vi "HFRR ADV v10.vi"() -> ()   [LabVIEW 2025] (continued)
              n2118 = Fract/Exp String To Number(string=w2526) -> (number=w2523:dbl)  [unwired: 3 in, 1 out]
              n2119 = Add(x=w2523, y=0.0) -> (x+y=w2521:dbl)
            }
            n2120 = String To Path(string=w2366) -> (path=w2464:path)
            n2121 = String To Path(string=w2364) -> (path=w2458:path)
            n2122 = local read "Numeric 11"() -> (w2448:i32)
            n2123 = local read "Numeric 13"() -> (w2450:i32)
            n2124 = Open/Create/Replace File "Open File"(file path (use dialog)=w2464) -> (refnum out=w2462:refnum<file>, error out=w2461:errorcluster)  [unwired: 5 in, 1 out]
            n2125 = Open/Create/Replace File "Open File"(file path (use dialog)=w2458) -> (refnum out=w2457:refnum<file>, error out=w2456:errorcluster)  [unwired: 5 in, 1 out]
            n2126 = for {
              N: w2448 -> [_]
              tunnel: w2462 -> [w2577]
              tunnel: w2461 -> [w2576]
              tunnel: [w2566] -> w2428 mode=indexing
              tunnel: [w2564] -> w2426 mode=indexing
              tunnel: [w2565] -> w2421 mode=indexing
              tunnel: w2447 -> [_]
              tunnel: [w2558] -> w2423 mode=indexing
              tunnel: [w2554] -> w2399 mode=indexing
              tunnel: [w2550] -> w2374 mode=indexing
              tunnel: [w2546] -> w2355 mode=indexing
              tunnel: [w2541] -> w2313 mode=indexing
              (unwired) TRUE ("line mode (F)")
              n2127 = Read from Text File "Read File"(file (use dialog)=w2577, error in=w2576) -> (text=w2542:string)  [unwired: 2 in, 3 out]
              n2128 = local write "String 7"(w2542) -> ()
              n2129 = String Subset(string=w2542, offset (0)=85, length (rest)=9 ("length (rest)")) -> (substring=w2545:string)
              n2130 = String Subset(string=w2542, offset (0)=35, length (rest)=9 ("length (rest)")) -> (substring=w2567:string)
              n2131 = String Subset(string=w2542, offset (0)=55, length (rest)=9 ("length (rest)")) -> (substring=w2553:string)
              n2132 = String Subset(string=w2542, offset (0)=25, length (rest)=9 ("length (rest)")) -> (substring=w2547:string)
              n2133 = String Subset(string=w2542, offset (0)=45, length (rest)=9 ("length (rest)")) -> (substring=w2555:string)
              n2134 = String Subset(string=w2542, offset (0)=0, length (rest)=14 ("length (rest)")) -> (substring=w2570:string)
              n2135 = String Subset(string=w2542, offset (0)=15, length (rest)=9 ("length (rest)")) -> (substring=w2573:string)
              n2136 = String Subset(string=w2542, offset (0)=65, length (rest)=9 ("length (rest)")) -> (substring=w2559:string)
              n2137 = Fract/Exp String To Number(string=w2545) -> (number=w2541:dbl)  [unwired: 3 in, 1 out]
              n2138 = Fract/Exp String To Number(string=w2567) -> (number=w2565:dbl)  [unwired: 3 in, 1 out]
              n2139 = Fract/Exp String To Number(string=w2553) -> (number=w2550:dbl)  [unwired: 3 in, 1 out]
              n2140 = Fract/Exp String To Number(string=w2547) -> (number=w2546:dbl)  [unwired: 3 in, 1 out]
              n2141 = Fract/Exp String To Number(string=w2555) -> (number=w2554:dbl)  [unwired: 3 in, 1 out]
              n2142 = Fract/Exp String To Number(string=w2570) -> (number=w2566:dbl)  [unwired: 3 in, 1 out]
              n2143 = Fract/Exp String To Number(string=w2573) -> (number=w2564:dbl)  [unwired: 3 in, 1 out]
              n2144 = Fract/Exp String To Number(string=w2559) -> (number=w2562:dbl)  [unwired: 3 in, 1 out]
              n2145 = Add(x=w2562, y=0.0) -> (x+y=w2558:dbl)
            }
            n2146 = for {
              N: w2450 -> [_]
              tunnel: w2457 -> [w2505]
              tunnel: w2456 -> [w2504]
              tunnel: [w2494] -> w2410 mode=indexing
              tunnel: [w2493] -> w2403 mode=indexing
              tunnel: w2447 -> [_]
              tunnel: [w2482] -> w2408 mode=indexing
              tunnel: [w2487] -> w2405 mode=indexing
              tunnel: [w2483] -> w2395 mode=indexing
              tunnel: [w2478] -> w2370 mode=indexing
              tunnel: [w2474] -> w2351 mode=indexing
              tunnel: [w2469] -> w2311 mode=indexing
              (unwired) 1.0 ("x")
              (unwired) TRUE ("line mode (F)")
              n2147 = Read from Text File "Read File"(file (use dialog)=w2505, error in=w2504) -> (text=w2470:string)  [unwired: 2 in, 3 out]
              n2148 = local write "String 12"(w2470) -> ()
              n2149 = String Subset(string=w2470, offset (0)=85, length (rest)=9 ("length (rest)")) -> (substring=w2472:string)
              n2150 = String Subset(string=w2470, offset (0)=35, length (rest)=9 ("length (rest)")) -> (substring=w2495:string)
              n2151 = String Subset(string=w2470, offset (0)=55, length (rest)=9 ("length (rest)")) -> (substring=w2480:string)
              n2152 = String Subset(string=w2470, offset (0)=25, length (rest)=9 ("length (rest)")) -> (substring=w2476:string)
              n2153 = String Subset(string=w2470, offset (0)=45, length (rest)=9 ("length (rest)")) -> (substring=w2485:string)
              n2154 = String Subset(string=w2470, offset (0)=15, length (rest)=9 ("length (rest)")) -> (substring=w2501:string)
              n2155 = String Subset(string=w2470, offset (0)=0, length (rest)=14 ("length (rest)")) -> (substring=w2498:string)
              n2156 = String Subset(string=w2470, offset (0)=65, length (rest)=9 ("length (rest)")) -> (substring=w2488:string)
              n2157 = Fract/Exp String To Number(string=w2472) -> (number=w2469:dbl)  [unwired: 3 in, 1 out]
              n2158 = Fract/Exp String To Number(string=w2495) -> (number=w2493:dbl)  [unwired: 3 in, 1 out]
              n2159 = Fract/Exp String To Number(string=w2480) -> (number=w2478:dbl)  [unwired: 3 in, 1 out]
              n2160 = Fract/Exp String To Number(string=w2476) -> (number=w2474:dbl)  [unwired: 3 in, 1 out]
              n2161 = Fract/Exp String To Number(string=w2485) -> (number=w2483:dbl)  [unwired: 3 in, 1 out]
              n2162 = Fract/Exp String To Number(string=w2501) -> (number=w2482:dbl)  [unwired: 3 in, 1 out]
              n2163 = Fract/Exp String To Number(string=w2498) -> (number=w2494:dbl)  [unwired: 3 in, 1 out]
              n2164 = Fract/Exp String To Number(string=w2488) -> (number=w2491:dbl)  [unwired: 3 in, 1 out]
              n2165 = Add(x=w2491, y=0.0) -> (x+y=w2487:dbl)
            }
            n2166 = Delete From Array(array=w2353, index=0) -> (array with subset deleted=w2326:dbl[])  [unwired: 1 in, 1 out]
            n2167 = Delete From Array(array=w2416, index=0) -> (array with subset deleted=w2389:dbl[])  [unwired: 1 in, 1 out]
            n2168 = Delete From Array(array=w2396, index=0) -> (array with subset deleted=w2384:dbl[])  [unwired: 1 in, 1 out]
            n2169 = Delete From Array(array=w2414, index=0) -> (array with subset deleted=w2415:dbl[])  [unwired: 1 in, 1 out]
            n2170 = call-poly <vilib>:"Mean.vi"("X"=w2326) -> ("mean"=→"КОФ2 4":dbl)  [unwired: 1 out]
            n2171 = call-poly <vilib>:"Mean.vi"("X"=w2389) -> ("mean"=→"КОФ3":dbl)  [unwired: 1 out]
            n2172 = call-poly <vilib>:"Mean.vi"("X"=w2384) -> ("mean"=→"CP3":dbl)  [unwired: 1 out]
            n2173 = Delete From Array(array=w2378, index=0) -> (array with subset deleted=w2305:dbl[])  [unwired: 1 in, 1 out]
            n2174 = Delete From Array(array=w2317, index=0) -> (array with subset deleted=w2304:dbl[])  [unwired: 1 in, 1 out]
            n2175 = Delete From Array(array=w2357, index=0) -> (array with subset deleted=w2328:dbl[])  [unwired: 1 in, 1 out]
            n2176 = Delete From Array(array=w2435, index=0) -> (array with subset deleted=w2390:dbl[])  [unwired: 1 in, 1 out]
            n2177 = Delete From Array(array=w2401, index=0) -> (array with subset deleted=w2386:dbl[])  [unwired: 1 in, 1 out]
            "array w/ subset deleted" <- w2386
            n2178 = Delete From Array(array=w2432, index=0) -> (array with subset deleted=w2433:dbl[])  [unwired: 1 in, 1 out]
            n2179 = call-poly <vilib>:"Mean.vi"("X"=w2328) -> ("mean"=→"КОФ2 2":dbl)  [unwired: 1 out]
            n2180 = call-poly <vilib>:"Mean.vi"("X"=w2390) -> ("mean"=→"КОФ1":dbl)  [unwired: 1 out]
            n2181 = Bundle "Bundle"(w2305, w2304) -> (w2310:cluster{dbl[], dbl[]})  [unwired: 1 in]
            n2182 = Bundle "Bundle"(w2305, w2433) -> (w2297:cluster{dbl[], dbl[]})  [unwired: 1 in]
            n2183 = Delete From Array(array=w2312, index=0) -> (array with subset deleted=w2300:dbl[])  [unwired: 1 in, 1 out]
            n2184 = Delete From Array(array=w2313, index=0) -> (array with subset deleted=w2302:dbl[])  [unwired: 1 in, 1 out]
            n2185 = Delete From Array(array=w2423, index=0) -> (array with subset deleted=w2424:dbl[])  [unwired: 1 in, 1 out]
            n2186 = Delete From Array(array=w2311, index=0) -> (array with subset deleted=w2298:dbl[])  [unwired: 1 in, 1 out]
            n2187 = Delete From Array(array=w2405, index=0) -> (array with subset deleted=w2406:dbl[])  [unwired: 1 in, 1 out]
            n2188 = Delete From Array(array=w2430, index=0) -> (array with subset deleted=w2336:dbl[])  [unwired: 1 in, 1 out]
            n2189 = Delete From Array(array=w2376, index=0) -> (array with subset deleted=w2332:dbl[])  [unwired: 1 in, 1 out]
            n2190 = Delete From Array(array=w2412, index=0) -> (array with subset deleted=w2334:dbl[])  [unwired: 1 in, 1 out]
            n2191 = Delete From Array(array=w2372, index=0) -> (array with subset deleted=w2330:dbl[])  [unwired: 1 in, 1 out]
            n2192 = Delete From Array(array=w2421, index=0) -> (array with subset deleted=w2335:dbl[])  [unwired: 1 in, 1 out]
            n2193 = Delete From Array(array=w2374, index=0) -> (array with subset deleted=w2331:dbl[])  [unwired: 1 in, 1 out]
            n2194 = Delete From Array(array=w2355, index=0) -> (array with subset deleted=w2327:dbl[])  [unwired: 1 in, 1 out]
            n2195 = Delete From Array(array=w2399, index=0) -> (array with subset deleted=w2385:dbl[])  [unwired: 1 in, 1 out]
            n2196 = Delete From Array(array=w2426, index=0) -> (array with subset deleted=w2387:dbl[])  [unwired: 1 in, 1 out]
            n2197 = Delete From Array(array=w2403, index=0) -> (array with subset deleted=w2333:dbl[])  [unwired: 1 in, 1 out]
            n2198 = Delete From Array(array=w2370, index=0) -> (array with subset deleted=w2329:dbl[])  [unwired: 1 in, 1 out]
            n2199 = Delete From Array(array=w2351, index=0) -> (array with subset deleted=w2325:dbl[])  [unwired: 1 in, 1 out]
            n2200 = Delete From Array(array=w2395, index=0) -> (array with subset deleted=w2383:dbl[])  [unwired: 1 in, 1 out]
            n2201 = Delete From Array(array=w2408, index=0) -> (array with subset deleted=w2388:dbl[])  [unwired: 1 in, 1 out]
            n2202 = Delete From Array(array=w2418, index=0) -> (array with subset deleted=w2301:dbl[])  [unwired: 1 in, 1 out]
            n2203 = Delete From Array(array=w2428, index=0) -> (array with subset deleted=w2303:dbl[])  [unwired: 1 in, 1 out]
            n2204 = Delete From Array(array=w2410, index=0) -> (array with subset deleted=w2299:dbl[])  [unwired: 1 in, 1 out]
            n2205 = Bundle "Bundle"(w2305, w2336) -> (w2323:cluster{dbl[], dbl[]})  [unwired: 1 in]
            n2206 = Bundle "Bundle"(w2305, w2390) -> (w2324:cluster{dbl[], dbl[]})  [unwired: 1 in]
            n2207 = Bundle "Bundle"(w2336, w2332) -> (w2338:cluster{dbl[], dbl[]})  [unwired: 1 in]
            n2208 = Bundle "Bundle"(w2301, w2300) -> (w2308:cluster{dbl[], dbl[]})  [unwired: 1 in]
            n2209 = Bundle "Bundle"(w2334, w2330) -> (w2340:cluster{dbl[], dbl[]})  [unwired: 1 in]
            n2210 = Bundle "Bundle"(w2301, w2334) -> (w2444:cluster{dbl[], dbl[]})  [unwired: 1 in]
            n2211 = Bundle "Bundle"(w2301, w2330) -> (w2368:cluster{dbl[], dbl[]})  [unwired: 1 in]
            n2212 = Bundle "Bundle"(w2301, w2389) -> (w2454:cluster{dbl[], dbl[]})  [unwired: 1 in]
            n2213 = Bundle "Bundle"(w2301, w2384) -> (w2392:cluster{dbl[], dbl[]})  [unwired: 1 in]
            n2214 = Bundle "Bundle"(w2301, w2415) -> (w2439:cluster{dbl[], dbl[]})  [unwired: 1 in]
            n2215 = Bundle "Bundle"(w2335, w2331) -> (w2339:cluster{dbl[], dbl[]})  [unwired: 1 in]
            n2216 = Bundle "Bundle"(w2303, w2302) -> (w2309:cluster{dbl[], dbl[]})  [unwired: 1 in]
            n2217 = Bundle "Bundle"(w2303, w2335) -> (w2446:cluster{dbl[], dbl[]})  [unwired: 1 in]
            n2218 = Bundle "Bundle"(w2303, w2331) -> (w2369:cluster{dbl[], dbl[]})  [unwired: 1 in]
            n2219 = Bundle "Bundle"(w2303, w2385) -> (w2393:cluster{dbl[], dbl[]})  [unwired: 1 in]
            n2220 = Bundle "Bundle"(w2303, w2387) -> (w2455:cluster{dbl[], dbl[]})  [unwired: 1 in]
            n2221 = Bundle "Bundle"(w2303, w2424) -> (w2437:cluster{dbl[], dbl[]})  [unwired: 1 in]
            n2222 = Bundle "Bundle"(w2333, w2329) -> (w2341:cluster{dbl[], dbl[]})  [unwired: 1 in]
            n2223 = Bundle "Bundle"(w2299, w2298) -> (w2307:cluster{dbl[], dbl[]})  [unwired: 1 in]
            n2224 = Bundle "Bundle"(w2299, w2333) -> (w2445:cluster{dbl[], dbl[]})  [unwired: 1 in]
            n2225 = Bundle "Bundle"(w2299, w2329) -> (w2367:cluster{dbl[], dbl[]})  [unwired: 1 in]
            n2226 = Bundle "Bundle"(w2299, w2383) -> (w2391:cluster{dbl[], dbl[]})  [unwired: 1 in]
            n2227 = Bundle "Bundle"(w2299, w2388) -> (w2453:cluster{dbl[], dbl[]})  [unwired: 1 in]
            n2228 = Bundle "Bundle"(w2299, w2406) -> (w2438:cluster{dbl[], dbl[]})  [unwired: 1 in]
            n2229 = call-poly <vilib>:"Mean.vi"("X"=w2386) -> ("mean"=→"CP1":dbl)  [unwired: 1 out]
            n2230 = call-poly <vilib>:"Mean.vi"("X"=w2327) -> ("mean"=→"КОФ2 3":dbl)  [unwired: 1 out]
            n2231 = call-poly <vilib>:"Mean.vi"("X"=w2385) -> ("mean"=→"CP2":dbl)  [unwired: 1 out]
            n2232 = call-poly <vilib>:"Mean.vi"("X"=w2387) -> ("mean"=→"КОФ2":dbl)  [unwired: 1 out]
            n2233 = call-poly <vilib>:"Mean.vi"("X"=w2325) -> ("mean"=→"КОФ2 5":dbl)  [unwired: 1 out]
            n2234 = call-poly <vilib>:"Mean.vi"("X"=w2383) -> ("mean"=→"CP4":dbl)  [unwired: 1 out]
            n2235 = call-poly <vilib>:"Mean.vi"("X"=w2388) -> ("mean"=→"КОФ4":dbl)  [unwired: 1 out]
            n2236 = Bundle "Bundle"(w2305, w2332) -> (w2296:cluster{dbl[], dbl[]})  [unwired: 1 in]
            n2237 = Bundle "Bundle"(w2305, w2386) -> (w2319:cluster{dbl[], dbl[]})  [unwired: 1 in]
            n2238 = Build Array "Build Array"(w2296, w2319) -> (w2322:cluster{dbl[], dbl[]}[])
            "XY Graph 17" <- w2322
            n2239 = Build Array "Build Array"(w2310, w2309, w2308, w2307) -> (→"Frequency ( Hz )":cluster{dbl[], dbl[]}[])
            n2240 = Build Array "Build Array"(w2338, w2339, w2340, w2341) -> (→"Air Temp ( °C ) vs Humidity ( % RH )":cluster{dbl[], dbl[]}[])
            n2241 = Build Array "Build Array"(w2323, w2446, w2444, w2445) -> (→"Air Temperature  ( °C )":cluster{dbl[], dbl[]}[])
            n2242 = Build Array "Build Array"(w2296, w2369, w2368, w2367) -> (→"Humidity ( %RH )":cluster{dbl[], dbl[]}[])
            n2243 = Build Array "Build Array"(w2324, w2455, w2454, w2453) -> (→"Coefficient Of Friction":cluster{dbl[], dbl[]}[])
            n2244 = Build Array "Build Array"(w2319, w2393, w2392, w2391) -> (→"Sample Temperature ( °C )":cluster{dbl[], dbl[]}[])
            n2245 = Build Array "Build Array"(w2297, w2437, w2439, w2438) -> (→"XY Graph 13":cluster{dbl[], dbl[]}[])
            n2246 = Bundle "Bundle"(w2305, w2328) -> (w2350:cluster{dbl[], dbl[]})  [unwired: 1 in]
            n2247 = Bundle "Bundle"(w2301, w2326) -> (w2348:cluster{dbl[], dbl[]})  [unwired: 1 in]
            n2248 = Bundle "Bundle"(w2303, w2327) -> (w2349:cluster{dbl[], dbl[]})  [unwired: 1 in]
            n2249 = Bundle "Bundle"(w2299, w2325) -> (w2347:cluster{dbl[], dbl[]})  [unwired: 1 in]
            n2250 = Build Array "Build Array"(w2350, w2349, w2348, w2347) -> (→"Stroke ( mm )":cluster{dbl[], dbl[]}[])
            n2251 = local write "XY Graph 16"(w2322) -> ()
          }
          frame #2 {
          }
          frame #3 {
            n2252 = local write "Numeric 8"(0 ("Numeric 8")) -> ()
            n2253 = local write "Numeric 11"(0 ("Numeric 11")) -> ()
            n2254 = local write "Numeric 12"(0 ("Numeric 12")) -> ()
            n2255 = local write "Numeric 13"(0 ("Numeric 13")) -> ()
            n2256 = property on="OPEN" class="Bool (strict)"("Visible"=TRUE) -> ()  [unwired: 2 in, 2 out]
            n2257 = local read "String Control 2"() -> (w2622:string)
            n2258 = local read "String Control 4"() -> (w2621:string)
            n2259 = local read "String Control 6"() -> (w2620:string)
            n2260 = local read "String Control 8"() -> (w2619:string)
            n2261 = Match Pattern(string=w2622, regular expression="Samples / cycle :- ") -> (after substring=w2636:string)  [unwired: 1 in, 3 out]
            n2262 = Match Pattern(string=w2622, regular expression="Frequency :- ") -> (after substring=w2655:string)  [unwired: 1 in, 3 out]
            n2263 = Match Pattern(string=w2621, regular expression="Samples / cycle :- ") -> (after substring=w2632:string)  [unwired: 1 in, 3 out]
            n2264 = Match Pattern(string=w2621, regular expression="Frequency :- ") -> (after substring=w2650:string)  [unwired: 1 in, 3 out]
            n2265 = Match Pattern(string=w2620, regular expression="Samples / cycle :- ") -> (after substring=w2628:string)  [unwired: 1 in, 3 out]
            n2266 = Match Pattern(string=w2620, regular expression="Frequency :- ") -> (after substring=w2645:string)  [unwired: 1 in, 3 out]
            n2267 = Match Pattern(string=w2619, regular expression="Samples / cycle :- ") -> (after substring=w2624:string)  [unwired: 1 in, 3 out]
            n2268 = Match Pattern(string=w2619, regular expression="Frequency :- ") -> (after substring=w2640:string)  [unwired: 1 in, 3 out]
            n2269 = String Subset(string=w2636, length (rest)=6 ("length (rest)")) -> (substring=w2638:string)  [unwired: 1 in]
            n2270 = String Subset(string=w2655, length (rest)=9 ("length (rest)")) -> (substring=w2657:string)  [unwired: 1 in]
            n2271 = String Subset(string=w2632, length (rest)=6 ("length (rest)")) -> (substring=w2634:string)  [unwired: 1 in]
            n2272 = String Subset(string=w2650, length (rest)=9 ("length (rest)")) -> (substring=w2652:string)  [unwired: 1 in]
            n2273 = String Subset(string=w2628, length (rest)=6 ("length (rest)")) -> (substring=w2630:string)  [unwired: 1 in]
            n2274 = String Subset(string=w2645, length (rest)=9 ("length (rest)")) -> (substring=w2647:string)  [unwired: 1 in]
            n2275 = String Subset(string=w2624, length (rest)=6 ("length (rest)")) -> (substring=w2626:string)  [unwired: 1 in]
            n2276 = String Subset(string=w2640, length (rest)=9 ("length (rest)")) -> (substring=w2642:string)  [unwired: 1 in]
            n2277 = Fract/Exp String To Number(string=w2638) -> (number=w2618:dbl)  [unwired: 3 in, 1 out]
            n2278 = Fract/Exp String To Number(string=w2657) -> (number=w2658:dbl)  [unwired: 3 in, 1 out]
            n2279 = Fract/Exp String To Number(string=w2634) -> (number=w2617:dbl)  [unwired: 3 in, 1 out]
            n2280 = Fract/Exp String To Number(string=w2652) -> (number=w2653:dbl)  [unwired: 3 in, 1 out]
            n2281 = Fract/Exp String To Number(string=w2630) -> (number=w2616:dbl)  [unwired: 3 in, 1 out]
            n2282 = Fract/Exp String To Number(string=w2647) -> (number=w2648:dbl)  [unwired: 3 in, 1 out]
            n2283 = Fract/Exp String To Number(string=w2626) -> (number=w2615:dbl)  [unwired: 3 in, 1 out]
            n2284 = Fract/Exp String To Number(string=w2642) -> (number=w2643:dbl)  [unwired: 3 in, 1 out]
            n2285 = local write "sample1"(w2618) -> ()
            n2286 = local write "freq1"(w2658) -> ()
            n2287 = local write "sample2"(w2617) -> ()
            n2288 = local write "freq2"(w2653) -> ()
            n2289 = local write "sample3"(w2616) -> ()
            n2290 = local write "freq3"(w2648) -> ()
            n2291 = local write "sample4"(w2615) -> ()
            n2292 = local write "freq 4"(w2643) -> ()
          }
        }
      }
    }
    n2293 = case shown="True" w2105 {
      selector: w2105 -> [_ w2234]
      frame False {
      }
      frame True {
        n2294 = Not(x=w2234) -> (.not. x?=w2230:bool)
        n2295 = local write "service 3"(w2230) -> ()
        n2296 = local write "OPEN 6"(w2230) -> ()
        n2297 = call <vilib>:"System Exec.vi"("wait until completion? (T)"=TRUE, "command line"="C:\\LAB-IQ\\Scar View.exe") -> ("error out"=→"error out 5":errorcluster)  [unwired: 6 in, 3 out]
      }
    }
    n2298 = case shown="\"Acquire\", Default" w2117 {
      frame "Acquire", Default {
        w3157 = 0.2 ("y")
        w3162 = 1.0 ("y")
        w3163 = 0.8 ("y")
        # "Elapsed time\ncof\nstroke\nAir temp\nTemp\nHumidity"
        n2299 = disable-structure shown="Disabled" {
          frame Disabled {
            n2300 = local read "Flag"() -> (w3180:dbl)
            n2301 = local read "RUN"() -> (w3177:bool)
            n2302 = Not(x=w3177) -> (.not. x?=w3176:bool)
            n2303 = Equal?(x=w3180, y=10.0) -> (x = y?=w3178:bool)
            n2304 = And(x=w3178, y=w3176) -> (x .and. y?=w3175:bool)
            n2305 = case shown="True" w3175 {
              frame False {
              }
              frame True {
                w3181 = FALSE ("Heater Button")
                n2306 = local write "Humidity"(w3181) -> ()
                n2307 = local write "Heater Button"(w3181) -> ()
              }
            }
          }
          frame Enabled {
          }
        }
        n2308 = disable-structure shown="Disabled" {
          frame Disabled {
            n2309 = case shown="True" {
              selector: _ -> [_ _]
              frame False {
              }
              frame True {
                w3272 = TRUE ("Heater")
                n2310 = local write "Humidity"(w3272) -> ()
                n2311 = local write "Heater Button"(w3272) -> ()
                n2312 = local read "TEST STANDARD"() -> (w3275:T3)
                n2313 = local read "TEST STANDARD"() -> (w3270:T3)
                n2314 = Equal?(x=w3275, y=enum16{"ASTM D6079", "ISO 12156", "Custom"}."ISO 12156" ("Test Standard")) -> (x = y?=w3273:bool)
                n2315 = Equal?(x=w3270, y=enum16{"ASTM D6079", "ISO 12156", "Custom"}."ASTM D6079" ("Test Standard")) -> (x = y?=w3269:bool)
                n2316 = case shown="True" w3273 {
                  frame False {
                  }
                  frame True {
                    n2317 = local write "Heater"(TRUE ("Heater")) -> ()
                    n2318 = local write "airtempflg"(FALSE ("airtempflg")) -> ()
                  }
                }
                n2319 = case shown="True" w3269 {
                  frame False {
                  }
                  frame True {
                    n2320 = local write "Heater"(FALSE ("Heater")) -> ()
                    n2321 = local write "airtempflg"(TRUE ("airtempflg")) -> ()
                  }
                }
              }
            }
          }
          frame Enabled {
          }
        }
        n2322 = stacked-sequence {
          frame #0 {
            n2323 = case shown="True" "RST FF" {
              frame False {
              }
              frame True {
                w3338 = 0.0 ("X Scale.Range:Maximum")
                n2324 = property on="Frictional Force ( N )" class="WFChart (strict)"("XScale.Maximum"=600.0 ("X Scale.Range:Maximum"), "XScale.Minimum"=w3338, "YScale.Maximum"=10.0 ("Y Scale.Range:Maximum"), "YScale.Minimum"=w3338) -> ()  [unwired: 2 in, 2 out]
              }
            }
          }
          frame #1 {
            n2325 = case shown="True" "RST TEMP" {
              frame False {
              }
              frame True {
                n2326 = property on="Temperature ( Deg C )" class="WFChart (strict)"("XScale.Minimum"=0.0 ("X Scale.Range:Minimum"), "XScale.Maximum"=600.0 ("X Scale.Range:Maximum"), "YScale.Minimum"=0.0 ("Y Scale.Range:Minimum"), "YScale.Maximum"=100.0 ("Y Scale.Range:Maximum")) -> ()  [unwired: 2 in, 2 out]
              }
            }
          }
          frame #2 {
            n2327 = case shown="True" "RSTCOF" {
              frame False {
              }
              frame True {
                n2328 = property on="Coefficient of Friction" class="WFChart (strict)"("XScale.Minimum"=0.0 ("X Scale.Range:Minimum"), "XScale.Maximum"=600.0 ("X Scale.Range:Maximum"), "YScale.Maximum"=1.0 ("X Scale.Range:Minimum"), "YScale.Minimum"=0.0 ("X Scale.Range:Minimum")) -> ()  [unwired: 2 in, 2 out]
              }
            }
          }
          frame #3 {
            n2329 = case shown="True" "RSTCOF 2" {
              frame False {
              }
              frame True {
                (unwired) 100.0 ("Y Scale.Range:Maximum")
                (unwired) 0.0 ("Y Scale.Range:Minimum")
                (unwired) 600.0 ("X Scale.Range:Maximum")
                (unwired) 0.0 ("X Scale.Range:Minimum")
              }
            }
          }
          frame #4 {
            n2330 = case shown="True" "RSTCOF 3" {
              frame False {
              }
              frame True {
                n2331 = property on="Electrical Contact Resistance ( % )" class="WFChart (strict)"("XScale.Minimum"=0.0 ("X Scale.Range:Minimum"), "XScale.Maximum"=600.0 ("X Scale.Range:Maximum"), "YScale.Minimum"=0.0 ("Y Scale.Range:Minimum"), "YScale.Maximum"=100.0 ("Y Scale.Range:Maximum")) -> ()  [unwired: 2 in, 2 out]
              }
            }
          }
        }
        n2332 = disable-structure shown="Disabled" {
          frame Disabled {
            n2333 = case shown="True" {
              selector: _ -> [_ _]
              frame False {
              }
              frame True {
                n2334 = local read "zflag 2"() -> (w3239:dbl)
                n2335 = local read "yflag"() -> (w3241:dbl)
                n2336 = Equal?(x=w3241, y=2.0 ("tflag")) -> (x = y?=w3243:bool)
                n2337 = Equal?(x=w3239, y=3.0 ("tflag")) -> (x = y?=w3242:bool)
                n2338 = And(x=w3243, y=w3242) -> (x .and. y?=w3237:bool)
                n2339 = case shown="True" w3237 {
                  frame False {
                  }
                  frame True {
                    w3268 = 0.0 ("zflag")
                    n2340 = local write "zflag"(w3268) -> ()
                    n2341 = local write "zflag 2"(w3268) -> ()
                    n2342 = Delete(path (use dialog)=path "C:/LAB-IQ-NXT/WO 2449 TT.sig" ("file path (dialog if empty)")) -> (deleted path=w3267:path)  [unwired: 4 in, 2 out]
                    n2343 = Delete(path (use dialog)=path "C:/LAB-IQ-NXT/WO 2449 TRH.sig" ("file path (dialog if empty)")) -> (deleted path=w3262:path)  [unwired: 4 in, 2 out]
                    n2344 = local read "SEN.RUN HRS"() -> (w3254:dbl)
                    n2345 = local read "SENSOR TIME"() -> (w3252:dbl)
                    n2346 = call <vilib>:"compatOverwrite.vi"("overwrite (F)"=TRUE) -> ("overwrite?"=w3244:T26)
                    n2347 = call <vilib>:"compatOverwrite.vi"("overwrite (F)"=TRUE) -> ("overwrite?"=w3248:T26)
                    n2348 = local read "Total No. of Tests"() -> (w3255:dbl)
                    n2349 = Add(x=w3252, y=w3254) -> (x+y=w3253:dbl)
                    "SEN.RUN HRS" <- w3253
                    n2350 = Open/Create/Replace File(file path (use dialog)=w3267, operation (0:open)=w3244) -> (refnum out=w3245:refnum<file>, error out=w3246:errorcluster)  [unwired: 4 in, 1 out]
                    n2351 = Open/Create/Replace File(file path (use dialog)=w3262, operation (0:open)=w3248) -> (refnum out=w3249:refnum<file>, error out=w3250:errorcluster)  [unwired: 4 in, 1 out]
                    n2352 = Deny Access(4:w3246, 6:T24."deny none" ("deny mode (2)"), 7:w3245) -> (3:w3266:refnum<file>)  [unwired: 1 out]
                    n2353 = Deny Access(4:w3250, 6:T24."deny none" ("deny mode (2)"), 7:w3249) -> (3:w3258:refnum<file>)  [unwired: 1 out]
                    n2354 = Number To Decimal String(number=w3255) -> (decimal integer string=w3263:string)  [unwired: 1 in]
                    n2355 = Number To Decimal String(number=w3253) -> (decimal integer string=w3259:string)  [unwired: 1 in]
                    n2356 = Write to Binary File(file (use dialog)=w3266, data=w3263, 5:FALSE ("prepend array or string size? (T)")) -> ()  [unwired: 3 in, 3 out]
                    n2357 = Write to Binary File(file (use dialog)=w3258, data=w3259, 5:FALSE ("prepend array or string size? (T)")) -> ()  [unwired: 3 in, 3 out]
                  }
                }
              }
            }
          }
          frame Enabled {
          }
        }
        n2358 = local read "RUN"() -> (w3166:bool)
        n2359 = local read "run replace"() -> (w3170:bool)
        n2360 = local read "run replace"() -> (w3169:bool)
        n2361 = case shown="True" w3166 {
          frame False {
            n2362 = local write "run replace"(FALSE ("run replace")) -> ()
          }
          frame True {
            "run replace" <- TRUE ("run replace")
          }
        }
        n2363 = local read "RUN"() -> (w3174:bool)
        n2364 = local read "Set Temp"() -> (w3136:dbl)
        n2365 = local read "SetTemp"() -> (w3138:dbl)
        n2366 = case shown="False" w3174 {
          tunnel: [FALSE ("TEST RUNNING") TRUE ("TEST RUNNING")] -> w3173
          frame False {
            w3357 = 0.0 ("Flag")
            n2367 = local write "Elapsed time"(0.0 ("elapsedtime")) -> ()
            n2368 = local write "Time Remaining"(w3357) -> ()
            n2369 = local write "Flag"(w3357) -> ()
            n2370 = local write "Remaining Time"(w3357) -> ()
          }
          frame True {
            n2371 = local write "Flag"(10.0 ("Flag")) -> ()
          }
        }
        n2372 = case shown="False" w3170 {
          frame False {
            n2373 = local read "zflag"() -> (→"zflag 2":dbl)
            n2374 = local write "yflag"(2.0 ("tflag")) -> ()
            n2375 = local write "FLAG 4"(0.0 ("FLAG")) -> ()
          }
          frame True {
            n2376 = local write "yflag"(1.0 ("tflag")) -> ()
            n2377 = local write "zflag"(3.0 ("zflag")) -> ()
          }
        }
        n2378 = local read "acq 2"() -> (w3168:bool)
        n2379 = local read "AIR TEMP"() -> (w3131:dbl)
        n2380 = local read "Amb temp"() -> (w3135:dbl)
        n2381 = case shown="True" "Save & Continue" {
          frame False {
          }
          frame True {
            "acq 2" <- TRUE ("acq 2")
          }
        }
        n2382 = local read "Set Rh"() -> (w3137:dbl)
        n2383 = Add(x=w3138, y=w3163) -> (x+y=w3164:dbl)
        n2384 = Subtract(x=w3138, y=w3163) -> (x-y=w3165:dbl)
        n2385 = Add(x=w3136, y=w3157) -> (x+y=w3158:dbl)
        n2386 = Subtract(x=w3136, y=w3157) -> (x-y=w3159:dbl)
        n2387 = And(x=w3168, y=w3169) -> (x .and. y?=w3167:bool)
        n2388 = Greater Or Equal?(x=w3131, y=15.0) -> (x >= y?=w3132:bool)
        "powstat" <- w3132
        n2389 = local read "Humidity ( %RH )"() -> (w3134:dbl)
        n2390 = case shown="True" "Save & Continue" {
          frame False {
          }
          frame True {
            n2391 = while {
              tunnel: "0123456789abcdefghijklmnopqrstuvwxyzABCDEFGHIJKLMNOPQRSTUVWXYZ" ("string 2") -> [w3328]
              shift-right: [w3326] -> w3321
              shift-left: "" -> [w3325]
              i -> [w3335]
              stop <- w3334 stop-if-true
              n2392 = Random Number (0-1)() -> (number: 0 to 1=w3329:dbl)
              n2393 = Multiply(x=w3329, y=62.0) -> (x*y=w3331:dbl)
              n2394 = Decrement(x="Length") -> (x-1=w3324:i16)
              n2395 = To Word Integer(number=w3331) -> (16bit integer=w3332:i16)
              n2396 = String Subset(string=w3328, offset (0)=w3332, length (rest)=1 ("length (rest)")) -> (substring=w3327:string)
              n2397 = Greater Or Equal?(x=w3335, y=w3324) -> (x >= y?=w3334:bool)
              n2398 = Concatenate Strings(w3327, w3325) -> (w3326:string)
            }
            n2399 = local write "UUID"(w3321) -> ()
          }
        }
        n2400 = In Range and Coerce(upper limit=w3164, x=w3135, lower limit=w3165) -> (In Range?=w3154:bool)  [unwired: 1 out]
        n2401 = Add(x=w3137, y=w3162) -> (x+y=w3161:dbl)
        n2402 = Subtract(x=w3137, y=w3162) -> (x-y=w3160:dbl)
        n2403 = local read "TEMP"() -> (w3133:dbl)
        n2404 = case shown="True" "Save & Continue" {
          frame False {
          }
          frame True {
            n2405 = local read "Operator ID"() -> (w3677:string)
            n2406 = local read "FILE"() -> (w3683:string)
            n2407 = String Length(string=w3683) -> (length=w3681:i32)
            n2408 = String Length(string=w3677) -> (length=w3678:i32)
            n2409 = Greater?(x=w3681, y=0) -> (0:w3680:bool)
            n2410 = Greater?(x=w3678, y=0) -> (0:w3676:bool)
            n2411 = And(x=w3680, y=w3676) -> (x .and. y?=w3675:bool)
            n2412 = case shown="True" w3675 {
              frame False {
                n2413 = stacked-sequence {
                  frame #0 {
                    n2414 = One Button Dialog(message="Please Enter a File Name and Operator ID to save data !", button name ("OK")="Ok") -> ()  [unwired: 1 out]
                  }
                  frame #1 {
                    n2415 = local write "Save & Continue"(FALSE ("OK Button")) -> ()
                  }
                }
                n2416 = local write "Save & Continue"(FALSE ("OK Button")) -> ()
              }
              frame True {
                n2417 = stacked-sequence {
                  frame #0 {
                    n2418 = local read "FILE"() -> (w3689:string)
                    n2419 = call "file check.vi"("file name in"=w3689) -> ("file name out"=w3688:string)  [unwired: 9 in, 1 out]
                    n2420 = call <vilib>:"Application Directory.vi"() -> ("Application Directory"=w3699:path)
                    n2421 = Build Path(base path=w3699, name or relative path="data") -> (appended path=w3698:path)
                    n2422 = call <vilib>:"Trim Whitespace.vi"("string"=w3688) -> ("trimmed string"=w3696:string)  [unwired: 1 in]
                    n2423 = call <vilib>:"Trim Whitespace.vi"("string"=w3688) -> ("trimmed string"=w3697:string)  [unwired: 1 in]
                    n2424 = List Folder(path=w3698) -> (folder names=w3694:string[])  [unwired: 3 in, 3 out]
                    n2425 = Match Pattern(string=w3696, regular expression="_(") -> (before substring=w3693:string)  [unwired: 1 in, 3 out]
                    n2426 = for {
                      tunnel: w3694 -> [w3708] mode=indexing
                      tunnel: w3693 -> [w3706]
                      shift-right: [w3704] -> w3691
                      shift-left: bool[] [] -> [w3705]
                      n2427 = Match Pattern(string=w3708, regular expression="_(") -> (before substring=w3707:string)  [unwired: 1 in, 3 out]
                      n2428 = Equal?(x=w3707, y=w3706) -> (x = y?=w3703:bool)
                      n2429 = case shown="True" w3703 {
                        tunnel: w3703 -> [_ w3711]
                        tunnel: w3705 -> [w3710 w3713]
                        tunnel: [w3710 w3712] -> w3704
                        frame False {
                        }
                        frame True {
                          n2430 = Insert Into Array(array=w3713, new element=w3711) -> (w3712:bool[])  [unwired: 1 in]
                        }
                      }
                    }
                    n2431 = Equal?(x=w3694, y=w3693) -> (x = y?=w3702:bool[])
                    n2432 = Or Array Elements(Boolean array=w3702) -> (logical OR=w3701:bool)
                    n2433 = Array Size(array=w3691) -> (size(s)=w3690:i32)
                    n2434 = case shown="True" w3701 {
                      tunnel: w3697 -> [_ w3721]
                      tunnel: w3690 -> [_ w3714]
                      frame False {
                      }
                      frame True {
                        n2435 = Number To Decimal String(number=w3714) -> (decimal integer string=w3717:string)  [unwired: 1 in]
                        n2436 = Search/Split String(string=w3721, search string/char (-)="_(" ("regular expression")) -> (substring before match=w3719:string)  [unwired: 1 in, 2 out]
                        n2437 = Concatenate Strings(w3719, "_(" ("regular expression"), w3717, ")" ("regular expression")) -> (w3715:string)
                        n2438 = local write "FILE"(w3715) -> ()
                      }
                    }
                  }
                  frame #1 {
                    w3723 = 0.0
                    w3736 = cluster{"y":dbl, dbl, "y":dbl}[] [] ("History Data")
                    w3737 = FALSE ("Heater Button")
                    (unwired) ")!" ("string")
                    (unwired) ")" ("string")
                    w3735 = dbl[] [] ("History Data")
                    w3741 = "\r"
                    # "C:\\WinDucom\\Data\\"
                    # "C:\\LAB-IQ-NXT\\data"
                    n2439 = local write "Humidity ( %RH )"(w3723) -> ()
                    n2440 = local write "Frequency ( Hz )"(w3723) -> ()
                    n2441 = local write "Stroke 3"(w3723) -> ()
                    n2442 = local write "speedop"(0.0 ("PIDclk 2")) -> ()
                    n2443 = local write "Set Temp 2"(65.0 ("Set Temp 2")) -> ()
                    n2444 = local write "AIR TEMP"(w3723) -> ()
                    n2445 = local write "clk"(0.0 ("clk")) -> ()
                    n2446 = local write "Stroke 4"(w3723) -> ()
                    n2447 = local write "Stroke"(w3723) -> ()
                    n2448 = local write "COF 3"(w3723) -> ()
                    n2449 = local write "COF 2"(w3723) -> ()
                    n2450 = local write "TEMP"(w3723) -> ()
                    n2451 = local write "ecr 3"(w3723) -> ()
                    n2452 = local write "FF 3"(w3723) -> ()
                    n2453 = local write "FF 2"(w3723) -> ()
                    n2454 = property on="Humidity ( %RH )" class="WFChart (strict)"("History Data"=w3735) -> ()  [unwired: 2 in, 2 out]
                    n2455 = property on="Coefficient of Friction" class="WFChart (strict)"("History Data"=w3735) -> ()  [unwired: 2 in, 2 out]
                    n2456 = property on="Coefficient of Friction" class="WFChart (strict)"("History Data"=w3735) -> ()  [unwired: 2 in, 2 out]
                    n2457 = property on="Frictional Force ( N )" class="WFChart (strict)"("History Data"=w3735) -> ()  [unwired: 2 in, 2 out]
                    n2458 = property on="Electrical Contact Resistance ( % )" class="WFChart (strict)"("History Data"=w3735) -> ()  [unwired: 2 in, 2 out]
                    n2459 = property on="Electrical Contact Resistance ( % )" class="WFChart (strict)"("History Data"=w3735) -> ()  [unwired: 2 in, 2 out]
                    n2460 = property on="Temperature ( Deg C )" class="WFChart (strict)"("History Data"=w3735) -> ()  [unwired: 2 in, 2 out]
                    n2461 = property on="Frictional Force ( N )" class="WFChart (strict)"("History Data"=w3735) -> ()  [unwired: 2 in, 2 out]
                    n2462 = property on="Coefficient of Friction" class="WFChart (strict)"("History Data"=w3735) -> ()  [unwired: 2 in, 2 out]
                    n2463 = property on="Frictional Force ( N )" class="WFChart (strict)"("History Data"=w3735) -> ()  [unwired: 2 in, 2 out]
                    n2464 = property on="Electrical Contact Resistance ( % )" class="WFChart (strict)"("History Data"=w3735) -> ()  [unwired: 2 in, 2 out]
                    n2465 = property on="Temperature ( Deg C )" class="WFChart (strict)"("History Data"=w3735) -> ()  [unwired: 2 in, 2 out]
                    n2466 = property on="Humidity ( %RH )" class="WFChart (strict)"("History Data"=w3735) -> ()  [unwired: 2 in, 2 out]
                    n2467 = property on="Stroke ( mm )" class="WFChart (strict)"("History Data"=w3736) -> ()  [unwired: 2 in, 2 out]
                    n2468 = property on="Stroke ( mm )" class="WFChart (strict)"("History Data"=w3736) -> ()  [unwired: 2 in, 2 out]
                    n2469 = local write "Humidity"(w3737) -> ()
                    n2470 = local write "Heater Button"(w3737) -> ()
                    n2471 = local read "FILE"() -> (w3731:string)
                    n2472 = disable-structure shown="Enabled" {
                      disable-tunnel: [w3776 _] -> w3722
                      frame Enabled {
                        n2473 = local read "NORMAL LOAD"() -> (w3776:dbl)
                      }
                      frame Disabled {
                      }
                    }
                    n2474 = call "file check.vi"("file name in"=w3731) -> ("error out"=w3734:errorcluster, "file name out"=w3728:string)  [unwired: 9 in]
                    n2475 = call "FILE PATH CREATION.vi"("error in"=w3734, "FILE NAME :"=w3728) -> ("FILE OUT"=w3727:path)  [unwired: 8 in, 1 out]
                    n2476 = Concatenate Strings(w3728, ".dgf" ("Substring")) -> (w3733:string)
                    n2477 = Concatenate Strings(w3728, ".duf" ("Substring")) -> (w3729:string)
                    n2478 = Multiply(x=w3722, y=1.0) -> (x*y=w3755:dbl)
                    n2479 = Build Path(base path=w3727, name or relative path=w3733) -> (appended path=w3726:path)
                    n2480 = Build Path(base path=w3727, name or relative path=w3729) -> (appended path=w3725:path)
                    n2481 = Number To Fractional String(number=w3755, width (-)=i16 5, precision (6)=i16 2) -> (F-format string=w3763:string)  [unwired: 1 in]
                    n2482 = local read "Fuel Discription :"() -> (w3751:string)
                    n2483 = local read "Batch Ref Num :"() -> (w3739:string)
                    n2484 = Get Date/Time String(date format (0)=enum16{"short", "long", "abbreviated"}."short") -> (date string=w3774:string, time string=w3771:string)  [unwired: 2 in]
                    n2485 = local read "Remarks :"() -> (w3750:string)
                    n2486 = Concatenate Strings("Load :- " ("Substring"), w3763, " grams ," ("Substring")) -> (w3762:string)
                    n2487 = local read "String 41"() -> (w3742:string)
                    n2488 = Concatenate Strings(w3751) -> (w3752:string)
                    n2489 = Concatenate Strings(w3739) -> (w3738:string)
                    n2490 = Concatenate Strings("tested by") -> (w3746:string)
                    n2491 = Concatenate Strings("(" ("Substring"), w3774, ")" ("Substring"), w3771) -> (w3744:string)
                    "concatenated string" <- w3744
                    n2492 = Concatenate Strings(w3750, "," ("string")) -> (w3749:string)
                    n2493 = Concatenate Strings("  TIME;      COF;       STROKE;     AIR TEMP;  TEMP;  HUMIDITY;  ECR; PID-OUT; FREQUENCY" ("Substring"), "\r") -> (w3758:string)
                    n2494 = Concatenate Strings(w3742, w3741, "Fuel Discription :-" ("Substring"), w3752, w3741, w3762, w3741, "Batch Ref Num :-" ("Substring"), w3738, w3741, " Remarks :- " ("Substring"), w3749, w3741, " Date :- " ("Substring"), w3744, w3741, "Tested By :-" ("Substring"), w3746) -> (w3756:string)
                    "REMARKS" <- w3756
                    n2495 = call <vilib>:"Write Characters To File.vi"("append to file? (new file:F)"=FALSE, "character string"=w3758, "file path (dialog if empty)"=w3726) -> ()  [unwired: 2 in, 1 out]
                    n2496 = call <vilib>:"Write Characters To File.vi"("append to file? (new file:F)"=FALSE, "character string"=w3756, "file path (dialog if empty)"=w3725) -> ()  [unwired: 2 in, 1 out]
                  }
                  frame #2 {
                    n2497 = local write "Cycles elapsed"(0 ("Cycles elapsed")) -> ()
                    n2498 = local write "cyclecount"(0 ("cyclecount")) -> ()
                    n2499 = local write "Save & Continue"(FALSE ("OK")) -> ()
                    n2500 = local write "autostrtflg"(TRUE ("autostrtflg")) -> ()
                    n2501 = local write "Save"(FALSE ("Save")) -> ()
                    n2502 = Get Date/Time In Seconds() -> (seconds since 1Jan1904=w3781:timestamp)
                    n2503 = To Double Precision Float(number=w3781) -> (double precision float=w3780:dbl)
                    n2504 = local write "acq timer"(w3780) -> ()
                    n2505 = One Button Dialog(message="Please ensure sample is mounted properly and machine is ready in all aspects for testing !", button name ("OK")="Ok") -> ()  [unwired: 1 out]
                  }
                  frame #3 {
                    n2506 = stacked-sequence {
                      frame #0 {
                        n2507 = local write "Main Dashboard Buttons"(T1."Dashboard" ("Main Dashboard Buttons")) -> ()
                        n2508 = local write "Main Tab"(T2."Acquire" ("Main Tab")) -> ()
                      }
                      frame #1 {
                        n2509 = local write "EVENT LOG"("" ("EVENT LOG")) -> ()
                      }
                      frame #2 {
                        n2510 = Wait (ms)(milliseconds to wait=u32 50) -> ()  [unwired: 1 out]
                      }
                      frame #3 {
                        n2511 = disable-structure shown="Disabled" {
                          frame Disabled {
                            n2512 = local read "EVENT LOG"() -> (w3793:string)
                            n2513 = call "Event Log.vi"("Content"="Test Details", "EVENT LOG"=w3793) -> ("EVENT LOG"=w3792:string)  [unwired: 8 in, 1 out]
                            n2514 = local write "EVENT LOG"(w3792) -> ()
                          }
                          frame Enabled {
                          }
                        }
                      }
                      frame #4 {
                        n2515 = Wait (ms)(milliseconds to wait=u32 50) -> ()  [unwired: 1 out]
                      }
                      frame #5 {
                        n2516 = local read "FILE"() -> (w3795:string)
                        n2517 = Concatenate Strings("File Name :" ("Content"), w3795) -> (w3796:string)
                        n2518 = local read "EVENT LOG"() -> (w3799:string)
                        n2519 = call "Event Log.vi"("Content"=w3796, "EVENT LOG"=w3799) -> ("EVENT LOG"=w3798:string)  [unwired: 8 in, 1 out]
                        n2520 = local write "EVENT LOG"(w3798) -> ()
                      }
                      frame #6 {
                        n2521 = Wait (ms)(milliseconds to wait=u32 50) -> ()  [unwired: 1 out]
                      }
                      frame #7 {
                        n2522 = local read "Batch Ref Num :"() -> (w3801:string)
                        n2523 = Concatenate Strings("Batch Ref No :" ("Content"), w3801) -> (w3802:string)
                        n2524 = local read "EVENT LOG"() -> (w3805:string)
                        n2525 = call "Event Log.vi"("Content"=w3802, "EVENT LOG"=w3805) -> ("EVENT LOG"=w3804:string)  [unwired: 8 in, 1 out]
                        n2526 = local write "EVENT LOG"(w3804) -> ()
                      }
                      frame #8 {
                        n2527 = Wait (ms)(milliseconds to wait=u32 50) -> ()  [unwired: 1 out]
                      }
                      frame #9 {
                        n2528 = local read "tested by"() -> (w3807:string)
                        n2529 = Concatenate Strings("Tested By :" ("Content"), w3807) -> (w3808:string)
                        n2530 = local read "EVENT LOG"() -> (w3811:string)
                        n2531 = call "Event Log.vi"("Content"=w3808, "EVENT LOG"=w3811) -> ("EVENT LOG"=w3810:string)  [unwired: 8 in, 1 out]
                        n2532 = local write "EVENT LOG"(w3810) -> ()
                      }
                      frame #10 {
                        n2533 = Wait (ms)(milliseconds to wait=u32 50) -> ()  [unwired: 1 out]
                      }
                      frame #11 {
                        n2534 = local read "TEST STANDARD"() -> (w3814:T3)
                        n2535 = case shown="\"ASTM D6079\", Default" w3814 {
                          tunnel: ["ASTM D6079" "ISO 12156" "CEC F-096-A-06" "Custom"] -> w3813
                          frame "ASTM D6079", Default {
                          }
                          frame "ISO 12156" {
                          }
                          frame "CEC F-096-A-06" {
                          }
                          frame "Custom" {
                          }
                        }
                        n2536 = Concatenate Strings("Test Standard :" ("Content"), w3813) -> (w3815:string)
                        n2537 = local read "EVENT LOG"() -> (w3818:string)
                        n2538 = call "Event Log.vi"("Content"=w3815, "EVENT LOG"=w3818) -> ("EVENT LOG"=w3817:string)  [unwired: 8 in, 1 out]
                        n2539 = local write "EVENT LOG"(w3817) -> ()
                      }
                      frame #12 {
                        n2540 = Wait (ms)(milliseconds to wait=u32 50) -> ()  [unwired: 1 out]
                      }
                      frame #13 {
                        n2541 = local read "Fuel Discription :"() -> (w3824:string)
                        n2542 = Concatenate Strings("Fuel Description :" ("Content"), w3824) -> (w3825:string)
                        n2543 = local read "EVENT LOG"() -> (w3828:string)
                        n2544 = call "Event Log.vi"("Content"=w3825, "EVENT LOG"=w3828) -> ("EVENT LOG"=w3827:string)  [unwired: 8 in, 1 out]
                        n2545 = local write "EVENT LOG"(w3827) -> ()
                      }
                      frame #14 {
                        n2546 = Wait (ms)(milliseconds to wait=u32 50) -> ()  [unwired: 1 out]
                      }
                      frame #15 {
                        n2547 = local read "Remarks :"() -> (w3830:string)
                        n2548 = Concatenate Strings("Remarks :" ("Content"), w3830) -> (w3831:string)
                        n2549 = local read "EVENT LOG"() -> (w3834:string)
                        n2550 = call "Event Log.vi"("Content"=w3831, "EVENT LOG"=w3834) -> ("EVENT LOG"=w3833:string)  [unwired: 8 in, 1 out]
                        n2551 = local write "EVENT LOG"(w3833) -> ()
                      }
                      frame #16 {
                        n2552 = Wait (ms)(milliseconds to wait=u32 50) -> ()  [unwired: 1 out]
                      }
                      frame #17 {
                        n2553 = local read "Operator ID"() -> (w3836:string)
                        n2554 = Concatenate Strings("Operator ID :" ("Content"), w3836) -> (w3838:string)
                        n2555 = local read "EVENT LOG"() -> (w3840:string)
                        n2556 = call "Event Log.vi"("Content"=w3838, "EVENT LOG"=w3840) -> ("EVENT LOG"=w3839:string)  [unwired: 8 in, 1 out]
                        n2557 = local write "EVENT LOG"(w3839) -> ()
                      }
                      frame #18 {
                        n2558 = Wait (ms)(milliseconds to wait=u32 50) -> ()  [unwired: 1 out]
                      }
                      frame #19 {
                        n2559 = disable-structure shown="Disabled" {
                          frame Disabled {
                            n2560 = local read "EVENT LOG"() -> (w3844:string)
                            n2561 = call "Event Log.vi"("Content"="Test Parameter", "EVENT LOG"=w3844) -> ("EVENT LOG"=w3843:string)  [unwired: 8 in, 1 out]
                            n2562 = local write "EVENT LOG"(w3843) -> ()
                          }
                          frame Enabled {
                          }
                        }
                      }
                      frame #20 {
                        n2563 = Wait (ms)(milliseconds to wait=u32 50) -> ()  [unwired: 1 out]
                      }
                      frame #21 {
                        n2564 = local read "Set Hz"() -> (w3848:dbl)
                        n2565 = Number To Fractional String(number=w3848, precision (6)=i16 2) -> (F-format string=w3847:string)  [unwired: 2 in]
                        n2566 = Concatenate Strings("Set Frequency [Hz] :" ("Content"), w3847) -> (w3850:string)
                        n2567 = local read "EVENT LOG"() -> (w3852:string)
                        n2568 = call "Event Log.vi"("Content"=w3850, "EVENT LOG"=w3852) -> ("EVENT LOG"=w3851:string)  [unwired: 8 in, 1 out]
                        n2569 = local write "EVENT LOG"(w3851) -> ()
                      }
                      frame #22 {
                        n2570 = Wait (ms)(milliseconds to wait=u32 50) -> ()  [unwired: 1 out]
                      }
                      frame #23 {
                        n2571 = local read "NORMAL LOAD"() -> (w3855:dbl)
                        n2572 = Number To Fractional String(number=w3855, precision (6)=i16 2) -> (F-format string=w3856:string)  [unwired: 2 in]
                        n2573 = Concatenate Strings("Applied Load [grams] :" ("Content"), w3856) -> (w3858:string)
                        n2574 = local read "EVENT LOG"() -> (w3860:string)
                        n2575 = call "Event Log.vi"("Content"=w3858, "EVENT LOG"=w3860) -> ("EVENT LOG"=w3859:string)  [unwired: 8 in, 1 out]
                        n2576 = local write "EVENT LOG"(w3859) -> ()
                      }
                      frame #24 {
                        n2577 = Wait (ms)(milliseconds to wait=u32 50) -> ()  [unwired: 1 out]
                      }
                      frame #25 {
                        n2578 = local read "Set Strk"() -> (w3863:dbl)
                        n2579 = Number To Fractional String(number=w3863, precision (6)=i16 2) -> (F-format string=w3864:string)  [unwired: 2 in]
                        n2580 = Concatenate Strings("Set Stroke [mm] :" ("Content"), w3864) -> (w3866:string)
                        n2581 = local read "EVENT LOG"() -> (w3868:string)
                        n2582 = call "Event Log.vi"("Content"=w3866, "EVENT LOG"=w3868) -> ("EVENT LOG"=w3867:string)  [unwired: 8 in, 1 out]
                        n2583 = local write "EVENT LOG"(w3867) -> ()
                      }
                      frame #26 {
                        n2584 = Wait (ms)(milliseconds to wait=u32 50) -> ()  [unwired: 1 out]
                      }
                      frame #27 {
                        n2585 = local read "Set Temp"() -> (w3871:dbl)
                        n2586 = Number To Fractional String(number=w3871, precision (6)=i16 2) -> (F-format string=w3872:string)  [unwired: 2 in]
                        n2587 = Concatenate Strings("Set Temperature [deg C] :" ("Content"), w3872) -> (w3874:string)
                        n2588 = local read "EVENT LOG"() -> (w3876:string)
                        n2589 = call "Event Log.vi"("Content"=w3874, "EVENT LOG"=w3876) -> ("EVENT LOG"=w3875:string)  [unwired: 8 in, 1 out]
                        n2590 = local write "EVENT LOG"(w3875) -> ()
                      }
                      frame #28 {
                        n2591 = Wait (ms)(milliseconds to wait=u32 50) -> ()  [unwired: 1 out]
                      }
                      frame #29 {
                        n2592 = local read "Set Rh"() -> (w3879:dbl)
                        n2593 = Number To Fractional String(number=w3879, precision (6)=i16 2) -> (F-format string=w3880:string)  [unwired: 2 in]
                        n2594 = Concatenate Strings("Set Humidity [%RH] :" ("Content"), w3880) -> (w3882:string)
                        n2595 = local read "EVENT LOG"() -> (w3884:string)
                        n2596 = call "Event Log.vi"("Content"=w3882, "EVENT LOG"=w3884) -> ("EVENT LOG"=w3883:string)  [unwired: 8 in, 1 out]
                        n2597 = local write "EVENT LOG"(w3883) -> ()
                      }
                      frame #30 {
                        n2598 = Wait (ms)(milliseconds to wait=u32 50) -> ()  [unwired: 1 out]
                      }
                      frame #31 {
                        n2599 = local read "test time"() -> (w3887:dbl)
                        n2600 = Number To Fractional String(number=w3887, precision (6)=i16 1) -> (F-format string=w3888:string)  [unwired: 2 in]
                        n2601 = Concatenate Strings("Test Duration [mins] :" ("Content"), w3888) -> (w3890:string)
                        n2602 = local read "EVENT LOG"() -> (w3892:string)
                        n2603 = call "Event Log.vi"("Content"=w3890, "EVENT LOG"=w3892) -> ("EVENT LOG"=w3891:string)  [unwired: 8 in, 1 out]
                        n2604 = local write "EVENT LOG"(w3891) -> ()
                      }
                      frame #32 {
                        w3893 = dbl[] [] ("History Data")
                        w3894 = cluster{"y":dbl, dbl, "y":dbl}[] [] ("History Data")
                        w3895 = FALSE ("Visible")
                        n2605 = property on="Stroke ( mm )" class="WFChart (strict)"("History Data"=w3894) -> ()  [unwired: 2 in, 2 out]
                        n2606 = property on="Humidity ( %RH )" class="WFChart (strict)"("History Data"=w3893) -> ()  [unwired: 2 in, 2 out]
                        n2607 = property on="Temperature ( Deg C )" class="WFChart (strict)"("History Data"=w3893) -> ()  [unwired: 2 in, 2 out]
                        n2608 = property on="Electrical Contact Resistance ( % )" class="WFChart (strict)"("History Data"=w3893) -> ()  [unwired: 2 in, 2 out]
                        n2609 = property on="Coefficient of Friction" class="WFChart (strict)"("History Data"=w3893) -> ()  [unwired: 2 in, 2 out]
                        n2610 = property on="Frictional Force ( N )" class="WFChart (strict)"("History Data"=w3893) -> ()  [unwired: 2 in, 2 out]
                        n2611 = property on="Coefficient of Friction" class="WFChart (strict)"("History Data"=w3893) -> ()  [unwired: 2 in, 2 out]
                        n2612 = property on="Frictional Force ( N )" class="WFChart (strict)"("History Data"=w3893) -> ()  [unwired: 2 in, 2 out]
                        n2613 = property on="Electrical Contact Resistance ( % )" class="WFChart (strict)"("History Data"=w3893) -> ()  [unwired: 2 in, 2 out]
                        n2614 = property on="Humidity ( %RH )" class="WFChart (strict)"("History Data"=w3893) -> ()  [unwired: 2 in, 2 out]
                        n2615 = property on="Stroke ( mm )" class="WFChart (strict)"("History Data"=w3894) -> ()  [unwired: 2 in, 2 out]
                        n2616 = property on="Temperature ( Deg C )" class="WFChart (strict)"("History Data"=w3893) -> ()  [unwired: 2 in, 2 out]
                        n2617 = property on="Service Password Log" class="Str"("Visible"=w3895) -> ()  [unwired: 2 in, 2 out]
                        n2618 = property on="Password 3" class="Clust (strict)"("Visible"=w3895) -> ()  [unwired: 2 in, 2 out]
                      }
                    }
                    "TEST FILE NAM,E SAVED" <- TRUE ("TEST FILE NAM,E SAVED")
                  }
                }
              }
            }
          }
        }
        n2619 = case shown="True" w3167 {
          frame False {
            n2620 = local write "tfalg"(0.0 ("tfalg")) -> ()
          }
          frame True {
            n2621 = local read "tfalg"() -> (w3312:dbl)
            n2622 = Equal?(x=w3312, y=0.0) -> (x = y?=w3313:bool)
            n2623 = case shown="True" w3313 {
              frame False {
              }
              frame True {
                n2624 = local read "Total No. of Tests"() -> (w3316:dbl)
                n2625 = local write "tfalg"(1.0 ("tfalg")) -> ()
                n2626 = local write "acq 2"(FALSE ("acq 2")) -> ()
                n2627 = Wait (ms)(milliseconds to wait=u32 200) -> ()  [unwired: 1 out]
                n2628 = Increment(x=w3316) -> (x+1=w3315:dbl)
                n2629 = local write "Total No. of Tests"(w3315) -> ()
              }
            }
          }
        }
        n2630 = local write "Test \nStatus"(w3173) -> ()
        n2631 = local write "st enable"(w3173) -> ()
        n2632 = local write "PWR"(w3173) -> ()
        n2633 = local write "Save"(w3173) -> ()
        n2634 = local read "Main Tab"() -> (w3130:T2)
        n2635 = case shown="True" w3154 {
          tunnel: [FALSE ("RUN") TRUE ("RUN")] -> w3153
          tunnel: [_ 1] -> w3146
          frame False {
          }
          frame True {
          }
        }
        n2636 = In Range and Coerce(upper limit=w3161, x=w3134, lower limit=w3160) -> (In Range?=w3152:bool)  [unwired: 1 out]
        n2637 = In Range and Coerce(upper limit=w3158, x=w3133, lower limit=w3159) -> (In Range?=w3150:bool)  [unwired: 1 out]
        n2638 = case shown="True" w3166 {
          frame False {
            n2639 = local read "Rt 3"() -> (w3294:bool)
            n2640 = case shown="True" w3294 {
              frame False {
              }
              frame True {
                n2641 = local write "Rt 3"(FALSE ("Rt 3")) -> ()
                n2642 = local write "Json End Flg"(TRUE ("Upld AR 2")) -> ()
              }
            }
            "Rt" <- TRUE ("Rt")
            "Rt 2" <- FALSE ("Rt")
          }
          frame True {
            n2643 = local read "Rt"() -> (w3301:bool)
            n2644 = local write "Rt 2"(TRUE ("Rt 2")) -> ()
            n2645 = case shown="True" w3301 {
              frame False {
              }
              frame True {
                w3302 = TRUE ("Upld AR 2")
                n2646 = local write "Rt"(FALSE ("Rt")) -> ()
                n2647 = local write "Upld AR"(w3302) -> ()
                n2648 = local write "Json St Flg"(w3302) -> ()
              }
